vi "12.4 MorphReconstruct-HDome.vi"() -> ()   [LabVIEW 2016]
doc: "This example shows how to use the Edge Tool in NI Vision. The Edge Tool finds edges (or sharp transitions in the pixels values) along a given line or ROI profile. The Edge Tool is a precursor function to many of the gauging and inspection tasks. For example, the location of the edges found along a line profile across an object can interpreted as the boundaries of the object whose dimensions have to be measured for a gauging application or the presence of a crack in the surface of an object for an inspection application."
uses:
  <vilib>/vision/NI_Vision_Development_Module.lvlib
panel:
  out "#of Items found":i32
  in  "Operation":enum32{"Dilate", "Erode"}(ring)
  in  "Tab":enum32{"Src ", "Marker", "H-Dome", "Results"}(tab)
  out "Src":T1(plugin-control)
  out "Marker":T1(plugin-control)
  out "HDome":T1(plugin-control)
  out "Result":T1(plugin-control)
  in  "Stop":bool
  # "Instruction:\nRun program, make sure the Dialate operation is selected.\n\nNote the H-Dome reconstruction can only work correctly when operation is Dilate for this case."
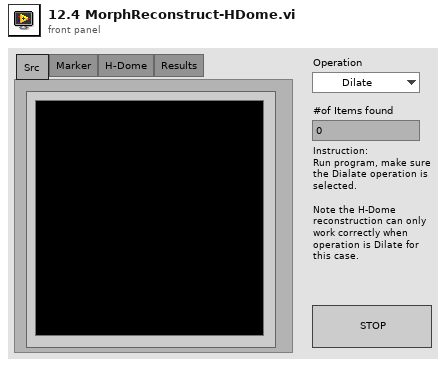
[diagram p1: front panel]
types:
  T1 = typedef "IMAQ Image.ctl" = refnum<image>
  T2 = enum16{"Bounding Box", "ID Label", "Center of Mass"}
  T3 = cluster{"Area":dbl, "Number of Holes":dbl, "Bounding Rect":cluster{"Left":dbl, "Top":dbl, "Right":dbl, "Bottom":dbl}, "Center of Mass":cluster{"X":dbl, "Y":dbl}, "Orientation":dbl, "Dimensions":cluster{"Width":dbl, "Height":dbl}}[]
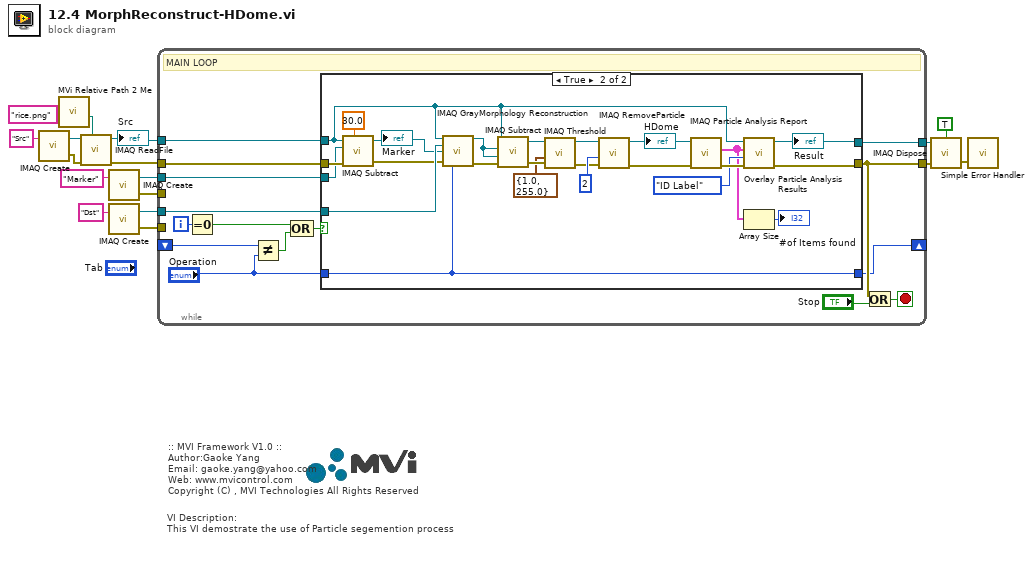
[diagram p0: block diagram]
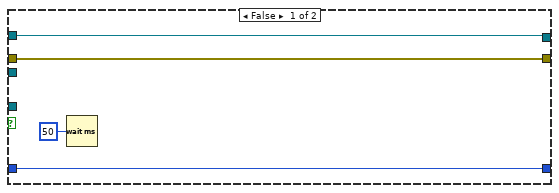
[diagram p2: hidden frame]
diagram:
  # "VI Description:\nThis VI demostrate the use of Particle segemention process"
  # ":: MVI Framework V1.0 ::\nAuthor:Gaoke Yang\nEmail: gaoke.yang@yahoo.com\nWeb: www.mvicontrol.com\nCopyright (C) , MVI Technologies All Rights Reserved"
  n1 = call "IMAQ Create"("Image Name"="Src") -> ("New Image"=w16:T1, "error out"=w15:errorcluster)  [unwired: 4 in]
  n2 = call "MVi Relative Path 2 Me.vi"("Relative Path"="rice.png" ("name or relative path")) -> ("Appended Dir"=w11:path)  [unwired: 5 in, 1 out]
  n3 = call "IMAQ ReadFile"("File Path"=w11, "error in (no error)"=w15, "Image"=w16) -> ("error out"=w5:errorcluster, "Image Out"=w4:T1)  [unwired: 4 in, 3 out]
  "Src" <- w4
  n4 = call "IMAQ Create"("Image Name"="Marker") -> ("New Image"=w8:T1, "error out"=w7:errorcluster)  [unwired: 4 in]
  n5 = call "IMAQ Create"("Image Name"="Dst") -> ("New Image"=w2:T1, "error out"=w1:errorcluster)  [unwired: 4 in]
  n6 = while "MAIN LOOP" {
    tunnel: w4 -> [w19]
    tunnel: w5 -> [w20]
    tunnel: [w29] -> w14
    tunnel: [w30] -> w13
    shift-right: [w26] -> _
    shift-left: _ -> [w24]
    tunnel: w8 -> [w21]
    tunnel: w7 -> [_]
    tunnel: w2 -> [w22]
    tunnel: w1 -> [_]
    i -> [w28]
    stop <- w31 stop-if-true
    # "MAIN LOOP"
    n7 = Equal To 0?(x=w28) -> (x = 0?=w25:bool)
    n8 = Not Equal?(x=w24, y="Operation") -> (x != y?=w23:bool)
    n9 = Compound Arithmetic op=OR(w25, w23) -> (w27:bool)
    n10 = case shown="True" w27 {
      tunnel: w20 -> [w36 w59]
      tunnel: [w34 w42] -> w30
      tunnel: [w36 w43] -> w29
      tunnel: [w35 w49] -> w26
      tunnel: "Operation" -> [w35 w49]
      tunnel: w22 -> [_ w60]
      tunnel: w21 -> [_ w50]
      tunnel: w19 -> [w34 w41]
      frame False {
        n11 = Wait (ms)(milliseconds to wait=u32 50) -> ()  [unwired: 1 out]
      }
      frame True {
        n12 = call "IMAQ Subtract"("Image Src A"=w41, "Constant"=30.0, "Image Dst"=w50, "error in (no error)"=w59) -> ("Image Dst Out"=w56:T1, "error out"=w57:errorcluster)  [unwired: 3 in]
        "Marker" <- w56
        n13 = call "IMAQ GrayMorphology Reconstruction"("Image Src"=w41, "Image Dst"=w60, "Image Marker"=w56, "error in (no error)"=w57, "Operation"=w49) -> ("Image Dst Out"=w55:T1, "error out"=w54:errorcluster)  [unwired: 9 in]
        n14 = call "IMAQ Subtract"("Image Src A"=w41, "Image Dst"=w55, "Image Src B"=w55, "error in (no error)"=w54) -> ("Image Dst Out"=w51:T1, "error out"=w53:errorcluster)  [unwired: 3 in]
        n15 = call "IMAQ Threshold"("error in (no error)"=w53, "Range"=cluster{"Lower value":sgl, "Upper value":sgl} {"Lower value"=1.0, "Upper value"=255.0}, "Image Src"=w51) -> ("error out"=w47:errorcluster, "Image Dst Out"=w46:T1)  [unwired: 3 in, 4 out]
        n16 = call "IMAQ RemoveParticle"("error in (no error)"=w47, "Number of Erosion"=2, "Image Src"=w46) -> ("error out"=w45:errorcluster, "Image Dst Out"=w37:T1)  [unwired: 4 in, 3 out]
        "HDome" <- w37
        n17 = call "IMAQ Particle Analysis Report"("error in (no error)"=w45, "Image"=w37) -> ("error out"=w44:errorcluster, "Particle Reports (Pixels)"=w39:T3)  [unwired: 1 in, 7 out]
        n18 = call "Overlay Particle Analysis Results.vi"("error in"=w44, "Overlay"=T2."ID Label", "Particle Reports (Pixels)"=w39, "Image"=w41) -> ("error out"=w43:errorcluster, "Image Out"=w42:T1)  [unwired: 6 in]
        "Result" <- w42
        n19 = Array Size(array=w39) -> (size(s)=→"#of Items found":i32)
      }
    }
    n20 = Or(x=w29, y="Stop") -> (x .or. y?=w31:bool)
  }
  n21 = call "IMAQ Dispose"("All Images? (No)"=TRUE, "Image"=w13, "error in (no error)"=w14) -> ("error out"=w10:errorcluster)  [unwired: 3 in]
  n22 = call <vilib>:"Simple Error Handler.vi"("error in (no error)"=w10) -> ()  [unwired: 4 in, 5 out]
